vi "Cursor Position to Cursor Index.vi"(9 "YScale.Ofst&Mult":T1, 10 "XScale.Ofst&Mult":T1, 11 "Cursor Position":T2) -> (3 "Index":cluster{"X index":i32, "Y index":i32})   [LabVIEW 2016]
uses:
  <vilib>/Utility/miscctls.llb/LVOffsetAndMultiplierTypeDef.ctl
  <vilib>/Utility/miscctls.llb/LVPointDoubleTypeDef.ctl
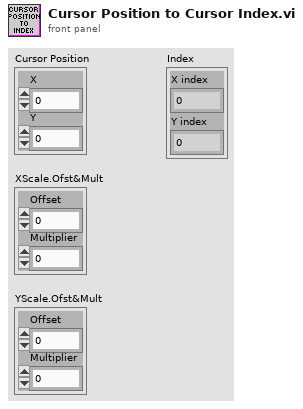
[diagram p1: front panel]
types:
  T1 = typedef "LVOffsetAndMultiplierTypeDef.ctl" = cluster{"Offset":dbl, "Multiplier":dbl}
  T2 = typedef "LVPointDoubleTypeDef.ctl" = cluster{"X":dbl, "Y":dbl}
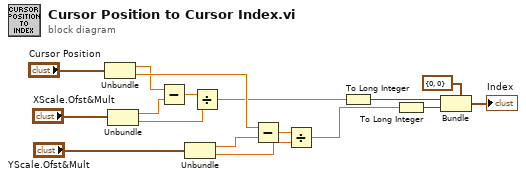
[diagram p0: block diagram]
diagram:
  n1 = Unbundle("Cursor Position") -> ("X"=w4:dbl, "Y"=w12:dbl)
  n2 = Unbundle("XScale.Ofst&Mult") -> ("Offset"=w7:dbl, "Multiplier"=w5:dbl)
  n3 = Subtract(x=w4, y=w7) -> (x-y=w6:dbl)
  n4 = Unbundle("YScale.Ofst&Mult") -> ("Offset"=w14:dbl, "Multiplier"=w15:dbl)
  n5 = Divide(x=w6, y=w5) -> (x/y=w2:dbl)
  n6 = Subtract(x=w12, y=w14) -> (x-y=w11:dbl)
  n7 = Divide(x=w11, y=w15) -> (x/y=w1:dbl)
  n8 = To Long Integer(number=w2) -> (32bit integer=w16:i32)
  n9 = To Long Integer(number=w1) -> (32bit integer=w3:i32)
  n10 = Bundle(cluster=cluster{"X index":i32, "Y index":i32} {"X index"=0, "Y index"=0}, "X index"=w16, "Y index"=w3) -> (→"Index":cluster{"X index":i32, "Y index":i32})
